vi "Limit.vi"(5 "Max":dbl=1.0, 7 "Min":dbl=-1.0, 11 "Input":dbl) -> (3 "Output":dbl)   [LabVIEW 2017]
doc: "Constrains the input to be between min and max"
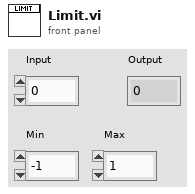
[diagram p1: front panel]
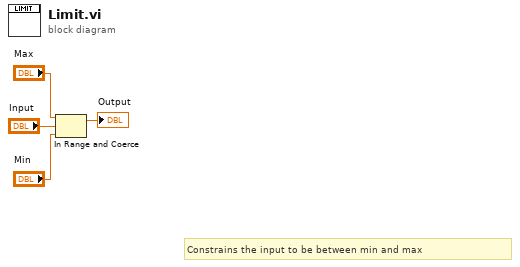
[diagram p0: block diagram]
diagram:
  # "Constrains the input to be between min and max"
  n1 = In Range and Coerce(upper limit="Max", x="Input", lower limit="Min") -> (coerced(x)=→"Output":dbl)  [unwired: 1 out]
